vi "Soft_Robot Model Two States.vi"() -> ()   [LabVIEW 2015]
uses:
  <vilib>/addons/Control Design/_Model Construction/Model Typedefs.llb/CD State Space Model (MIMO).ctl
  <vilib>/addons/Control Design/_Model Construction/Model Typedefs.llb/CD General Elements.ctl
  <vilib>/Platform/TimedLoop/XDataNode/timing_clust.ctl
  <vilib>/Platform/TimedLoop/XDataNode/nitl_modes.ctl
  <vilib>/Platform/TimedLoop/XDataNode/wakeup.ctl
  <vilib>/Analysis/7linalg.llb/Create Special Real Matrix.vi
  <vilib>/addons/Control Design/_Model Construction/Model Creation.llb/Model Creation SubVI/cd_Create State Space Model.vi
  <vilib>/addons/Control Design/_Stochastic Systems/Stochastic Systems.llb/CD Construct Noise Model (Numeric).vi
  <vilib>/addons/Control Design/_State Feedback Control/State Feedback Control.llb/State Feedback Control SubVis/cd_Discretized Linear Quadratic Regulator.vi
  <vilib>/Simulation/Estimation/Implementation/NILVSim Discrete Kalman Filter.llb/SIM Disc KF Pred and Corr with Pred Gain with Checking Direct LV.vi
  <vilib>/FPGAPlugInAG/myRIO-1900/niLvFpga_Open_myRIO-1900.vi
  <vilib>/rvi/interface/common/dynamic/niFpgaDynamicAddResources.vi
  <vilib>/Utility/error.llb/Error Cluster From Error Code.vi
  <vilib>/rvi/errors/niLvFpgaAdjustHostInterfaceError.vi
  <vilib>/FPGAPlugInAG/Dynamic/niLvFpga_Close_Dynamic.vi
  <vilib>/Platform/TimedLoop/XDataNode/XDataNode.xnode
  <vilib>/Simulation/Implementation/XNodeFramework/SimXNode/SimX.xnode
  <vilib>/rvi/interface/nirviOpenFPGA/nirviOpenFPGA.xnode
  FPGA Bitfiles/ACC20115_FPGATarget_CurrentControlle_Dt5vFgOzYtY.lvbitx
  Current Controller.vi
  <vilib>/rvi/interface/nirviReadWriteControl/nirviReadWriteControl.xnode
  <vilib>/rvi/interface/nirviCloseFPGA/nirviCloseFPGA.xnode
  <vilib>/addons/Control Design/_Model Construction/NI_LinSys_Model Creation.lvlib
  <vilib>/addons/Control Design/_State Feedback Control/NI_CD_State Feedback Control.lvlib
  <vilib>/addons/Control Design/_Stochastic Systems/NI_CD_Stochastic Systems.lvlib
  <vilib>/Analysis/NI_AALPro.lvlib
  <vilib>/Platform/TimedLoop/XDataNode/XDNodeRunTimeDep.lvlib
  NiFpgaLv.dll
  <vilib>/rvi/interface/Simulation/niFpgaSimulationCallBeginRW.vi
  <vilib>/addons/Control Design/_Model Construction/NI_LinSys_Model Typedefs.lvlib
panel:
  in  "SP1: 2":dbl(slide)=40.87020302841148 min=0.0 max=0.0 scale=0.0..720.0
  in  "Tab Control":enum32{"Outputs", "Inputs"}(tab)
  out "Fusion Data":dbl(graph)
  out "KF estimate":dbl[](graph)
  in  "Stop":bool
  out "DAC Inlet Valve 2":i32(graph)
  in  "Current (mA)":i32
  out "Status?":bool
  out "State-Space Model":T1 {"Transport Delay" format="%.2f"; "D" format="%#.2g"; "C" format="%#.2g"; "B" format="%#.2g"; "A" format="%#.2g"; "properties"."Sampling Time" format="%#.6p"; "properties"."Output Delays" format="%.4f"; "properties"."Input Delays" format="%.4f"}
  out "Kalman Filter Gain M(k)":dbl[][](array[numeric])
  in  "LQR Matrix (Q)":dbl[](array[slide])=[1.133823501217849, 15.19911082952933] scale=0.001..1000.0
  in  "LQR Output  matrix (R)":dbl[](array[slide])=[0.061359072734131735] scale=0.0001..10.0
  in  "xhat(0|-1)":dbl[](array[numeric])=[1.0, 0.0]
  in  "Cov P(0|-1)":dbl[][](array[numeric])=[[1.0, 0.0], [0.0, 1.0]]
  out "xhat(k|k)":dbl[](array[numeric])
  out "xhat(k+1|k)":dbl[](array[numeric])
  in  "A":dbl[][](array[numeric]) format="%#.5g"
  in  "B":dbl[][](array[numeric]) format="%#.5g"
  in  "C":dbl[][](array[numeric]) format="%#.5g"
  in  "KF Q":dbl[][](array[numeric])=[[0.01, 0.0], [0.0, 0.001]]
  in  "KF R":dbl[][](array[numeric])=[[0.1]]
  in  "E{v}":dbl[](array[numeric]) format="%#.2g"
  in  "E{w}":dbl[](array[numeric]) format="%#.2g"
  in  "G":dbl[][](array[numeric]) format="%#.2g"
  out "error out":errorcluster
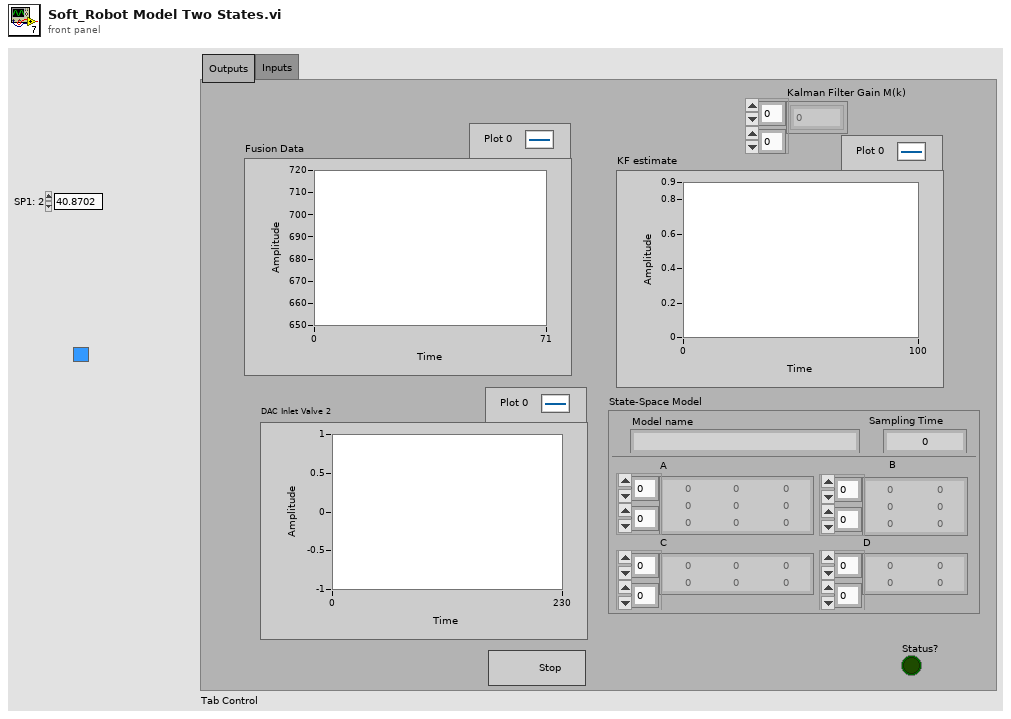
[diagram p1: front panel]
types:
  T1 = typedef "NI_LinSys_Model Typedefs.lvlib/CD State Space Model (MIMO).ctl" = cluster{"properties":T2, "A":dbl[][], "B":dbl[][], "C":dbl[][], "D":dbl[][], "StateNames":string[], "Transport Delay":dbl[][]}
  T2 = typedef "NI_LinSys_Model Typedefs.lvlib/CD General Elements.ctl" = cluster{"Model name":string, "Input names":string[], "Output names":string[], "Input Delays":dbl[], "Output Delays":dbl[], "Sampling Time":dbl, "Notes":string}
  T3 = typedef "XDNodeRunTimeDep.lvlib/timing_clust.ctl" = cluster{"Expected End [f-1]":u64, "Actual End [f-1]":u64, "Finished Late? [f-1]":bool, "Expected End [i-1]":u64, "Actual End [i-1]":u64, "Finished Late? [i-1]":bool, "Expected Start [i]":u64, "Actual Start [i]":u64, "Expected Start [f]":u64, "Actual Start [f]":u64, "Source Name":string, "Structure Name":string, "Period":i64, "Deadline":i64, "Offset":i64, "Start":i64, "Priority":i32, "Timeout":i32, "Mode":T4, "Wakeup Reason":T5, "Error":errorcluster, "Source Type":string, "Secondary Source Type":string, "Global End Time":u64, "Global Start Time":u64, "Frame Duration":u64, "Iteration Duration":u64, "Assigned CPU":i32, "I/O Scan Engine Mode":u32}
  T4 = typedef "XDNodeRunTimeDep.lvlib/nitl_modes.ctl" = enum32{"No Change", "Process missed periods, maintain original phase", "Discard missed periods, maintain original phase", "Process missed periods, ignore original phase", "Discard missed periods, ignore original phase"}
  T5 = typedef "XDNodeRunTimeDep.lvlib/wakeup.ctl" = enum32{"Normal", "Aborted", "Asynchronous wakeup", "Timing source error", "Timed loop error", "Timeout"}
  T6 = enum16{"state weighting", "output weighting, Dim Q = Ny", "output weighting, Dim Q = Nx"}
  T7 = enum32{"Identity", "Diagonal", "Toepliz", "Vandermonde", "Companion"}
  T8 = typedef "NI_Matrix.lvlib/RealMatrix.ctl" = dbl[][]
  T9 = typedef "NI_CD_Stochastic Systems.lvlib/cd_Stochastic State-Space Model.ctl" = cluster{"Sampling Time (s)":dbl, "G":dbl[][], "B":dbl[][], "A":dbl[][], "C":dbl[][], "D":dbl[][], "H":dbl[][]}
  T10 = typedef "NI_CD_Stochastic Systems.lvlib/cd_Second-Order Statistics Noise Model.ctl" = cluster{"Q":dbl[][], "E{w}":dbl[], "E{v}":dbl[], "R":dbl[][], "N":dbl[][]}
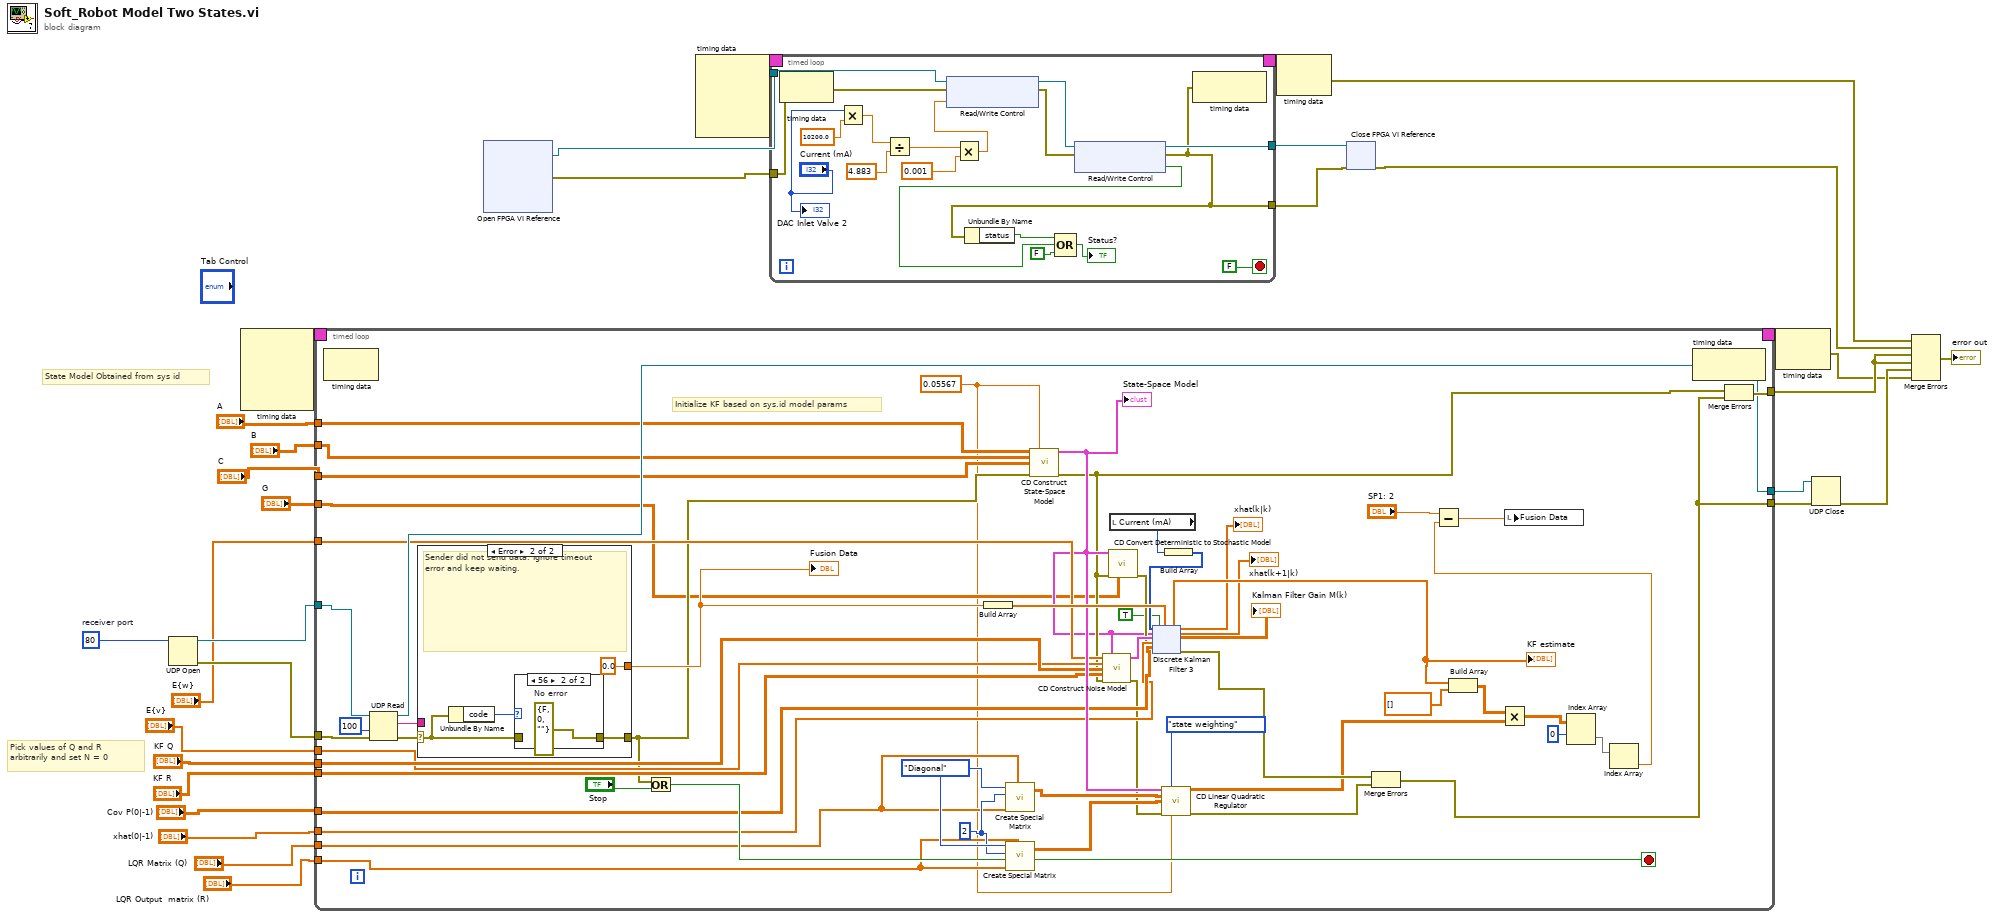
[diagram p0: block diagram]
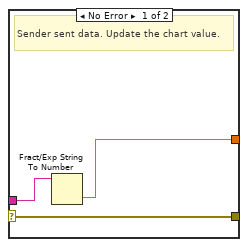
[diagram p2: hidden frame]
diagram:
  w29 = u16 80  # receiver port
  # "Pick values of Q and R\narbitrarily and set N = 0"
  # "State Model Obtained from sys id"
  n1 = UDP Open(11:w29) -> (port=w28:refnum<k16>, 0:w27:errorcluster)  [unwired: 4 in, 1 out]
  n2 = node-c288() -> (w11:T3)  [unwired: 4 in]
  n3 = timed-loop {
    tunnel: [w62] -> w24
    tunnel: w28 -> [w57]
    tunnel: w27 -> [w56]
    tunnel: [w53] -> w26
    tunnel: "A" -> [w52]
    tunnel: "B" -> [w51]
    tunnel: "C" -> [w50]
    tunnel: "KF Q" -> [w49]
    tunnel: "KF R" -> [w48]
    tunnel: "Cov P(0|-1)" -> [w47]
    tunnel: "xhat(0|-1)" -> [w46]
    tunnel: "E{v}" -> [w45]
    tunnel: "E{w}" -> [w44]
    tunnel: "LQR Matrix (Q)" -> [w35]
    tunnel: "LQR Output  matrix (R)" -> [w34]
    timing: w11 -> [_]
    timing-out: [_] -> w10
    tunnel: "G" -> [w38]
    tunnel: [w32] -> w2
    stop <- w54 stop-if-true
    w67 = 2
    w74 = T7."Diagonal" ("matrix type")
    w33 = 0.05567 ("Sampling Time (s)")
    # "Initialize KF based on sys.id model params"
    n4 = node-c288() -> ()  [unwired: 1 in, 1 out]
    n5 = UDP Read(connection ID=w57, timeout ms (25000)=100, 8:w56) -> (data out=w59:string, error out=w58:errorcluster, 3:w53:refnum<k16>)  [unwired: 3 out]
    n6 = case shown="Error" w58 {
      selector: w58 -> [w90 w94]
      tunnel: w59 -> [w91 _]
      tunnel: [w90 w93] -> w43
      tunnel: [w89 0.0] -> w55
      frame No Error {
        # "Sender sent data. Update the chart value."
        n7 = Fract/Exp String To Number(string=w91) -> (number=w89:dbl)  [unwired: 3 in, 1 out]
      }
      frame Error {
        # "Sender did not send data. Ignore timeout error and keep waiting."
        n8 = Unbundle By Name(w94) -> ("code"=w95:i32)
        n9 = case shown="56" w95 {
          tunnel: w94 -> [w96 _]
          tunnel: [w96 w97] -> w93
          frame Default {
          }
          frame 56 {
            w97 = errorcluster {"status"=FALSE, "code"=0, "source"=""}  # No error
          }
        }
      }
    }
    "Fusion Data" <- w55
    n10 = Or(x=w43, y="Stop") -> (x .or. y?=w54:bool)
    n11 = Build Array ("Build Array 6")(w55) -> (w78:dbl[])
    n12 = call-poly <vilib>:"Create Special Matrix.vi"("matrix type"=w74, "matrix size"=w67, "Input Vector1"=w35, "Input Vector2"=w35) -> ("Special Matrix"=w71:T8)  [unwired: 1 in, 1 out]
    n13 = call-poly <vilib>:"Create Special Matrix.vi"("matrix type"=w74, "matrix size"=w67, "Input Vector1"=w34, "Input Vector2"=w34) -> ("Special Matrix"=w70:T8)  [unwired: 1 in, 1 out]
    n14 = call-poly <vilib>:"CD Construct State-Space Model.vi"("A"=w52, "Sampling Time (s)"=w33, "B"=w51, "C"=w50, "error in (no error)"=w43) -> ("State-Space Model"=w72:T1, "error out"=w42:errorcluster)  [unwired: 9 in]
    "State-Space Model" <- w72
    n15 = call <vilib>:"CD Convert Deterministic to Stochastic Model.vi"("Deterministic State-Space Model"=w72, "error in (no error)"=w42, "G"=w38) -> ("Stochastic State-Space Model"=w39:T9, "error out"=w40:errorcluster)  [unwired: 11 in]
    n16 = call-poly <vilib>:"CD Construct Noise Model.vi"("E{w}"=w44, "Stochastic State-Space Model"=w39, "E{v}"=w45, "Q"=w49, "R"=w48, "error in (no error)"=w42) -> ("Second-Order Statistics Noise Model out"=w65:T10, "error out"=w41:errorcluster)  [unwired: 8 in]
    n17 = local read "Current (mA)"() -> (w79:i32)
    n18 = call-poly <vilib>:"CD Linear Quadratic Regulator.vi"("Continuous State-Space Model"=w72, "Weighting Type"=T6."state weighting", "Q"=w71, "R"=w70, "error in (no error)"=w41, "Sampling Time (s)"=w33) -> ("Optimal Gain (K)"=w69:dbl[][], "error out"=w68:errorcluster)  [unwired: 6 in, 2 out]
    n19 = Build Array ("Build Array 5")(w79) -> (w75:i32[])
    n20 = xnode ("Discrete Kalman Filter 3")("input u(k)"=w75, "Stochastic State-Space Model"=w39, "Second-Order Statistics Noise Model"=w65, "Initial State Estimate xhat(0|-1)"=w46, "Initial Estimation Error Covariance P(0|-1)"=w47, "Initialize?"=TRUE, "Output y(k)"=w78, "error in (no error)"=w40) -> ("Estimated Output yhat(k)"=w77:dbl[], "Corrected State Estimate xhat(k|k)"=→"xhat(k|k)":dbl[], "Predicted State Estimate xhat(k+1|k)"=→"xhat(k+1|k)":dbl[], "Kalman Filter Gain M(k)"=→"Kalman Filter Gain M(k)":dbl[][], "error out"=w76:errorcluster)  [unwired: 3 out]
    "KF estimate" <- w77
    n21 = Merge Errors(w76, w68) -> (w32:errorcluster)
    n22 = Build Array ("Build Array 9")(w77, dbl[] [] ("element")) -> (w82:dbl[][])
    n23 = Multiply(x=w82, y=w69) -> (x*y=w84:dbl[][])
    n24 = Index Array(array=w84, index (row)=0) -> (element=w86:dbl[])  [unwired: 1 in]
    n25 = Index Array ("Index Array 2")(array=w86) -> (element=w80:dbl)  [unwired: 1 in]
    n26 = Subtract(x="SP1: 2", y=w80) -> (x-y=w63:dbl)
    n27 = local write "Fusion Data"(w63) -> ()
    n28 = node-c288() -> ()  [unwired: 1 in, 1 out]
    n29 = Merge Errors(w42, w32) -> (w62:errorcluster)
  }
  n30 = xnode "Open FPGA VI Reference"() -> ("FPGA VI Reference Out"=w8:refnum<k20>, "error out"=w7:errorcluster)  [unwired: 2 in]
  n31 = node-c288() -> (w6:T3)  [unwired: 4 in]
  n32 = timed-loop {
    tunnel: w8 -> [w130]
    tunnel: w7 -> [w115]
    tunnel: [w114] -> w30
    tunnel: [w123] -> w31
    timing: w6 -> [_]
    timing-out: [_] -> w5
    stop <- FALSE stop-if-true
    n33 = node-c288() -> ()  [unwired: 1 in, 1 out]
    n34 = Multiply(x="Current (mA)", y=10200.0) -> (x*y=w118:dbl)
    n35 = Divide(x=w118, y=4.883) -> (x/y=w121:dbl)
    n36 = Multiply(x=w121, y=0.001) -> (x*y=w117:dbl)
    n37 = xnode "Read/Write Control"("FPGA VI Reference In"=w130, "error in"=w115, "DAC Inlet Valve"=w117) -> ("FPGA VI Reference Out"=w129:refnum<k20>, "error out"=w128:errorcluster)
    n38 = xnode "Read/Write Control"("FPGA VI Reference In"=w129, "error in"=w128) -> ("FPGA VI Reference Out"=w123:refnum<k20>, "error out"=w114:errorcluster, "Inlet Overflow?"=w124:bool)
    n39 = Unbundle By Name(w114) -> ("status"=w126:bool)
    n40 = Compound Arithmetic op=OR(w126, w124, FALSE ("value")) -> (→"Status?":bool)
    n41 = node-c288(w114) -> ()  [unwired: 1 out]
    "DAC Inlet Valve 2" <- "Current (mA)"
  }
  n42 = node-c288(w5) -> (w3:errorcluster)
  n43 = xnode "Close FPGA VI Reference"("FPGA VI Reference In"=w31, "error in"=w30) -> ("error out"=w4:errorcluster)
  n44 = node-c288(w10) -> (w1:errorcluster)
  n45 = UDP Close(connection ID=w26, 8:w2) -> (error out=w25:errorcluster)  [unwired: 1 out]
  n46 = Merge Errors(w3, w4, w24, w24, w25, w1) -> (→"error out":errorcluster)
